vi "Test.vi"() -> ()   [LabVIEW 2024]
uses:
  C:/Users/Andrey/Desktop/wpf_bounds_test/WpfBoundsTest/Release/WindowsFormsControlLibrary.dll
  WindowsFormsControlLibrary.dll
panel:
  in  "UserControl1":refnum<k24>(container)
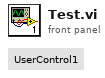
[diagram p1: front panel]
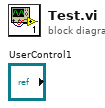
[diagram p0: block diagram]
diagram:
